vi "LVJSON Get.vi"(8 "error in (no error)":errorcluster, 10 "Root Path ([]=Root)":string[](array[string]), 11 "Root Element in":T1) -> (0 "error out":errorcluster, 1 "Element out":T1, 2 "Exists?":bool, 3 "dup Root Element":T1)   [LabVIEW 2019, in "labview_json.lvlib"]
uses:
  labview_json.lvlib
  Element.ctl
  Element Type.ctl
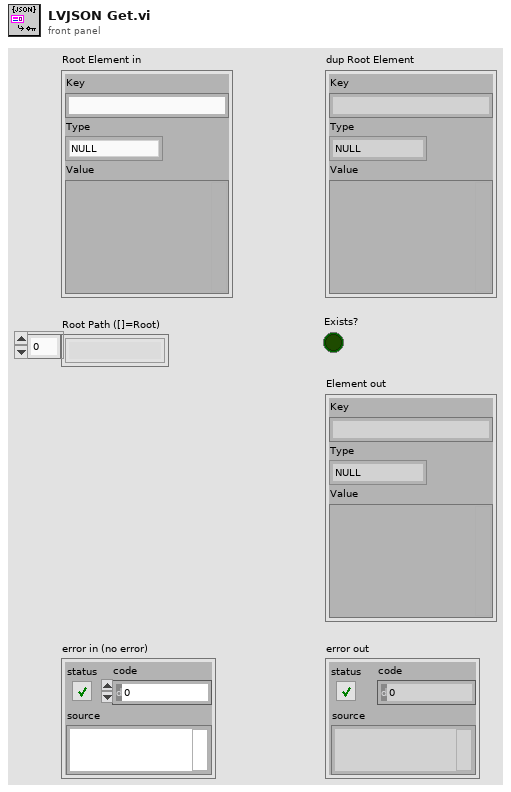
[diagram p1: front panel]
types:
  T1 = typedef "labview_json.lvlib/Element.ctl" = cluster{"Key":string, "Type":T2, "Value":variant}
  T2 = typedef "labview_json.lvlib/Element Type.ctl" = enum8{"NULL", "BOOL", "INT", "UINT", "FLOAT", "STRING", "ARRAY", "OBJECT", "SKIP"}
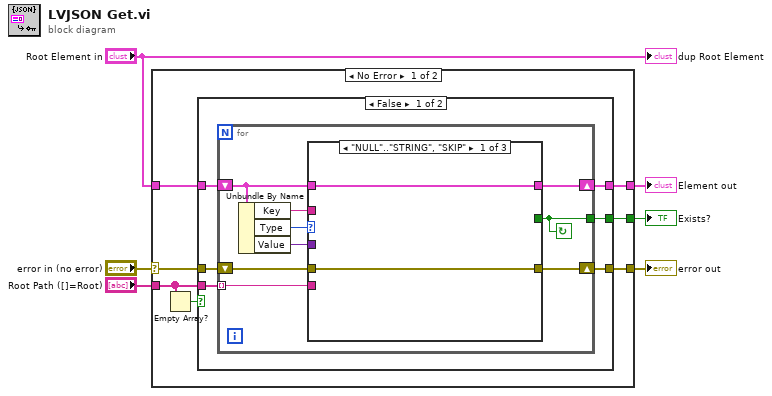
[diagram p0: block diagram]
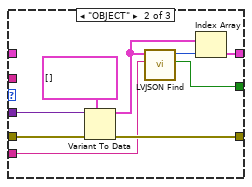
[diagram p2: hidden frame]
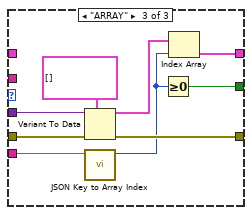
[diagram p3: hidden frame]
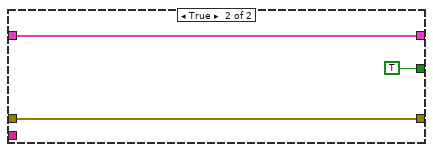
[diagram p4: hidden frame]
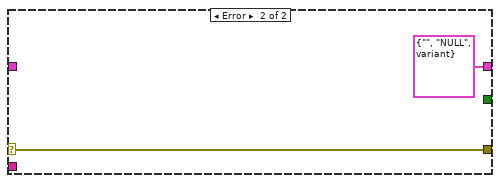
[diagram p5: hidden frame]
diagram:
  n1 = case shown="No Error" "error in (no error)" {
    selector: "error in (no error)" -> [w13 w53]
    tunnel: "Root Path ([]=Root)" -> [w8 _]
    tunnel: [w12 w53] -> w4
    tunnel: [w9 T1 {"Key"="", "Type"=enum."NULL", "Value"=variant} ("Root Element in")] -> w3
    tunnel: "Root Element in" -> [w11 _]
    tunnel: [w10 _] -> w2
    frame No Error {
      n2 = Empty Array?(array=w8) -> (empty?=w7:bool)
      n3 = case shown="False" w7 {
        tunnel: w8 -> [w19 _]
        tunnel: w13 -> [w18 w49]
        tunnel: [w17 w49] -> w12
        tunnel: w11 -> [w16 w51]
        tunnel: [w15 TRUE] -> w10
        tunnel: [w14 w51] -> w9
        frame False {
          n4 = for {
            tunnel: w19 -> [w20] mode=indexing
            shift-right: [w24] -> w17
            shift-left: w18 -> [w25]
            shift-right: [w23] -> w14
            shift-left: w16 -> [w22]
            tunnel: [w21] -> w15
            stop <- w21 continue-if-true
            n5 = Unbundle By Name(w22) -> ("Key"=w26:string, "Type"=w28:T2, "Value"=w27:variant)
            n6 = case shown="\"NULL\"..\"STRING\", \"SKIP\"" w28 {
              tunnel: w27 -> [_ w39 w48]
              tunnel: w26 -> [_ _ _]
              tunnel: w20 -> [_ w35 w41]
              tunnel: w25 -> [w30 w37 w46]
              tunnel: [w30 w36 w45] -> w24
              tunnel: [w29 w33 w43] -> w23
              tunnel: w22 -> [w29 _ _]
              tunnel: [_ w32 w42] -> w21
              frame "NULL".."STRING", "SKIP" {
              }
              frame "OBJECT" {
                n7 = Variant To Data(error in=w37, type=T1[] [] ("Values"), Variant=w39) -> (data=w34:T1[], error out=w36:errorcluster)
                n8 = call "LVJSON Find.vi"("Key"=w35, "Elements in"=w34) -> ("Found?"=w32:bool, "Index"=w31:i32)  [unwired: 8 in]
                n9 = Index Array(array=w34, index=w31) -> (element=w33:T1)
              }
              frame "ARRAY" {
                n10 = Variant To Data(error in=w46, type=T1[] [] ("Values"), Variant=w48) -> (data=w44:T1[], error out=w45:errorcluster)
                n11 = call "JSON Key to Array Index.vi"("Key"=w41) -> ("Index"=w40:i32)  [unwired: 8 in, 2 out]
                n12 = Greater Or Equal To 0?(x=w40) -> (x >= 0?=w42:bool)
                n13 = Index Array(array=w44, index=w40) -> (element=w43:T1)
              }
            }
          }
        }
        frame True {
        }
      }
    }
    frame Error {
    }
  }
  "error out" <- w4
  "Element out" <- w3
  "Exists?" <- w2
  "dup Root Element" <- "Root Element in"
